vi "Oscillator.vi"(4 "Sampling info":cluster{"Fs":dbl, "#s":dbl}={"Fs"=1000.0, "#s"=1000.0} {"Fs" format="%.2p"}, 6 "Sub Oscillator Type":T2, 7 "Waveform type":T1(ring), 8 "Error in":errorcluster, 9 "Pulse Width":dbl=50.0 format="%0.2f", 10 "Amplitude":dbl=1.0 format="%#_13g", 11 "Frequency":dbl=500.0 format="%#_13g") -> (0 "Error out":errorcluster, 3 "Waveform out":waveform(dbl)(graph))   [LabVIEW 2019]
uses:
  Type Definitions/Sub Oscillalator Type.ctl
  <vilib>/measure/NI_MABase.lvlib
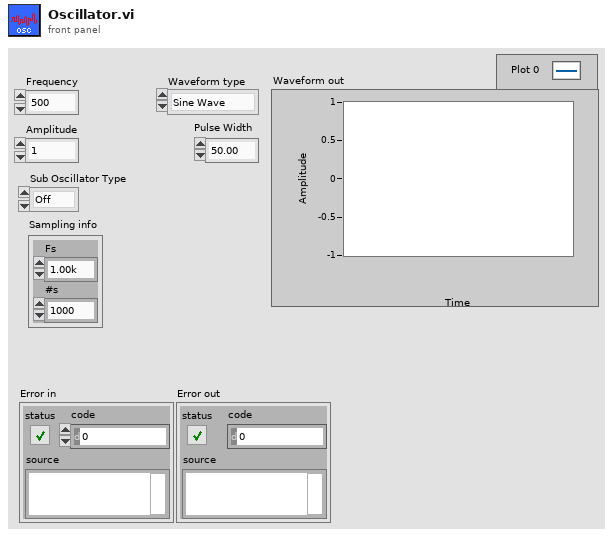
[diagram p1: front panel]
types:
  T1 = enum16{"Sine Wave", "Triangle Wave", "Square Wave", "Sawtooth Wave"}
  T2 = typedef "Sub Oscillalator Type.ctl" = enum16{"Off", "One Octave", "Two Octaves"}
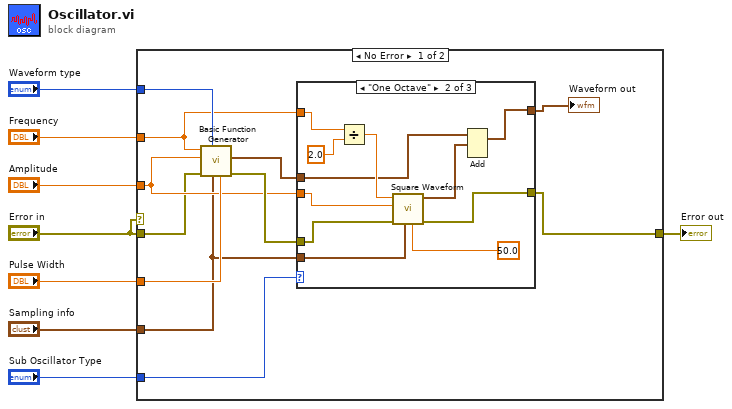
[diagram p0: block diagram]
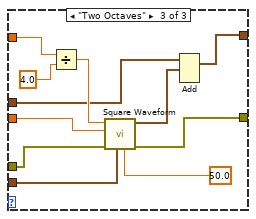
[diagram p3: hidden frame]
diagram:
  n1 = case shown="No Error" "Error in" {
    tunnel: "Waveform type" -> [w19 _]
    tunnel: "Pulse Width" -> [w16 _]
    tunnel: "Sub Oscillator Type" -> [w15 _]
    tunnel: "Frequency" -> [w14 _]
    tunnel: "Amplitude" -> [w13 _]
    tunnel: "Error in" -> [w12 w44]
    tunnel: "Sampling info" -> [w11 _]
    tunnel: [w10 w44] -> w1
    frame No Error {
      n2 = call <vilib>:"Basic Function Generator.vi"("square wave duty cycle (%)"=w16, "sampling info"=w11, "signal type"=w19, "error in (no error)"=w12, "amplitude"=w13, "frequency"=w14) -> ("error out"=w17:errorcluster, "signal out"=w18:waveform(dbl))  [unwired: 3 in, 1 out]
      n3 = case shown="\"One Octave\"" w15 {
        tunnel: w18 -> [w21 w26 w36]
        tunnel: w17 -> [w20 w32 w34]
        tunnel: [w21 w25 w38] -> w9
        tunnel: [w20 w23 w39] -> w10
        tunnel: w14 -> [_ w30 w37]
        tunnel: w13 -> [_ w28 w35]
        tunnel: w11 -> [_ w22 w33]
        frame "Off", Default {
        }
        frame "One Octave" {
          n4 = Divide(x=w30, y=2.0) -> (x/y=w27:dbl)
          n5 = call <vilib>:"Square Waveform.vi"("duty cycle (%)"=50.0, "sampling info"=w22, "error in (no error)"=w32, "amplitude"=w28, "frequency"=w27) -> ("error out"=w23:errorcluster, "signal out"=w24:waveform(dbl))  [unwired: 5 in]
          n6 = Add(1:w24, 2:w26) -> (0:w25:waveform(dbl))  [unwired: 1 in, 1 out]
        }
        frame "Two Octaves" {
          n7 = Divide(x=w37, y=4.0) -> (x/y=w42:dbl)
          n8 = call <vilib>:"Square Waveform.vi"("duty cycle (%)"=50.0, "sampling info"=w33, "error in (no error)"=w34, "amplitude"=w35, "frequency"=w42) -> ("error out"=w39:errorcluster, "signal out"=w43:waveform(dbl))  [unwired: 5 in]
          n9 = Add(1:w43, 2:w36) -> (0:w38:waveform(dbl))  [unwired: 1 in, 1 out]
        }
      }
      "Waveform out" <- w9
    }
    frame Error {
    }
  }
  "Error out" <- w1
